vi "qtest.vi"() -> ()   [LabVIEW 2020]
uses:
  5df3b76d-11be-4eb4-bfe8-7a0dabd50acf.vi
  7e36f1bc-8072-43ef-9e73-c82577f060f5.vi
panel:
  out "x-y":u32
  out "Elemente 5":cluster{"Numerisch":dbl, "Numerisch 2":dbl}[](array[cluster])
  out "Elemente 4":cluster{"Numerisch":dbl, "Numerisch 2":dbl}[](array[cluster])
  out "Elemente 3":cluster{"Numerisch":dbl, "Numerisch 2":dbl}[](array[cluster])
  in  "Stopp":bool
  out "Elemente 2":cluster{"Numerisch":dbl, "Numerisch 2":dbl}[](array[cluster])
  out "Elemente":cluster{"Numerisch":dbl, "Numerisch 2":dbl}[](array[cluster])
  in  "Cluster":cluster{"Numerisch":dbl, "Numerisch 2":dbl}
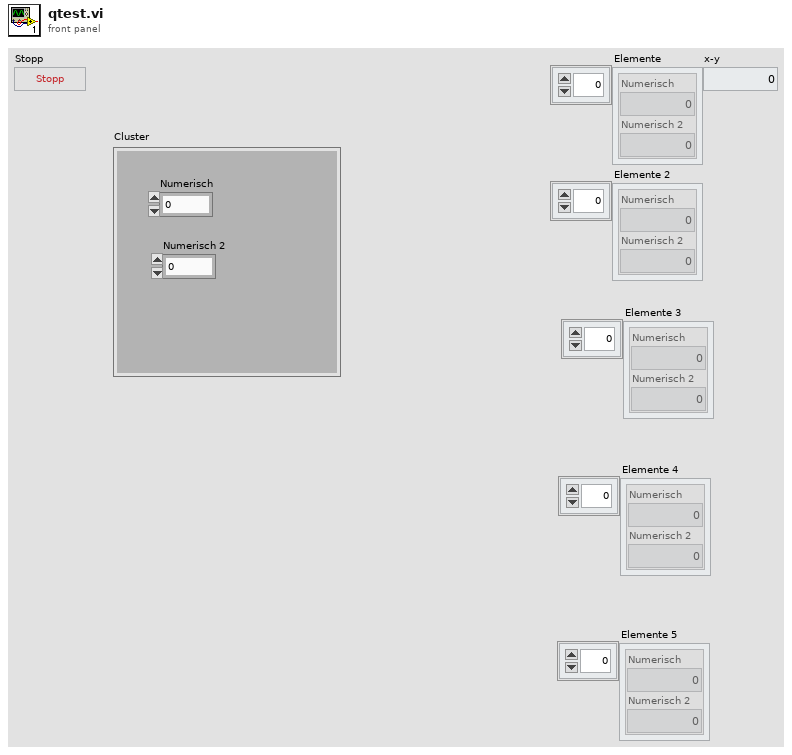
[diagram p1: front panel]
types:
  T1 = cluster{"number: 0 to 1":dbl, "number: 0 to 1":dbl}
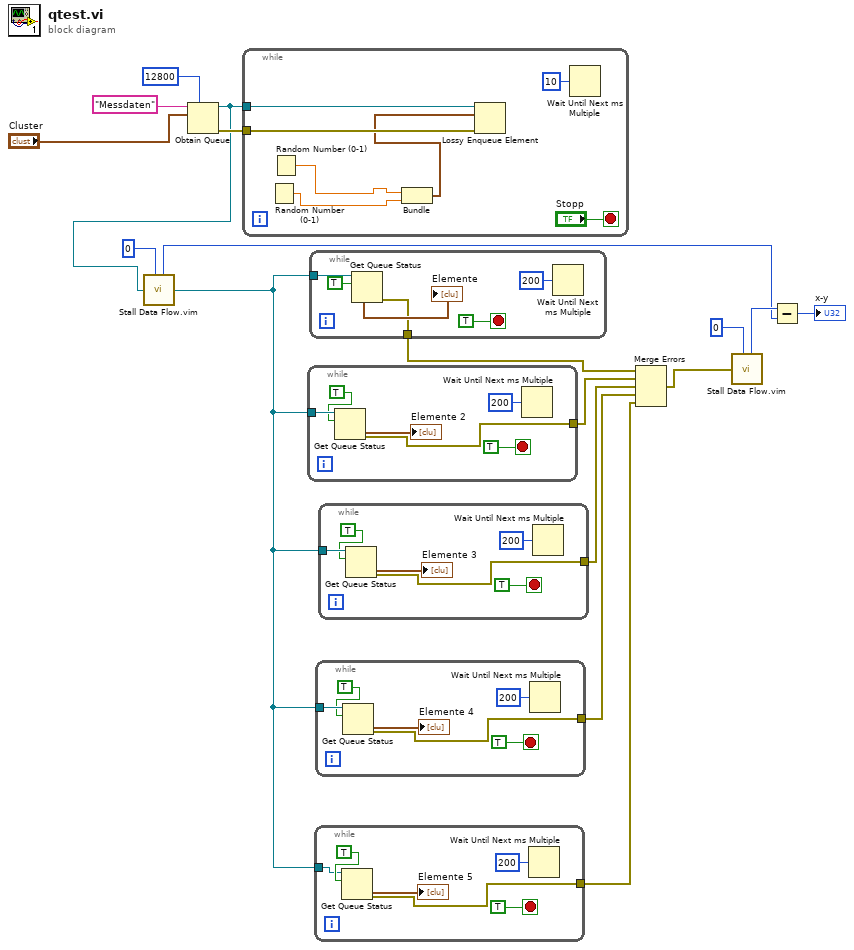
[diagram p0: block diagram]
diagram:
  n1 = Obtain Queue(max queue size (-1, unlimited)=12800 ("Maximale Queue-Größe (-1, unbegrenzt)"), name (unnamed)="Messdaten" ("Name (unbenannt)"), element data type="Cluster") -> (queue out=w8:refnum<queue>, error out=w15:errorcluster)  [unwired: 2 in, 1 out]
  n2 = call "Stall Data Flow.vim"("value in"=w8, "milliseconds to wait"=u32 0) -> ("millisecond timer value"=w2:u32, "value out"=w7:refnum<queue>)
  n3 = while {
    tunnel: w8 -> [w24]
    tunnel: w15 -> [w23]
    stop <- "Stopp" stop-if-true
    n4 = Random Number (0-1)() -> (number: 0 to 1=w21:dbl)
    n5 = Random Number (0-1)() -> (number: 0 to 1=w20:dbl)
    n6 = Bundle("number: 0 to 1"=w20, "number: 0 to 1"=w21) -> (w19:T1)  [unwired: 1 in]
    n7 = Lossy Enqueue Element(queue=w24, element=w19, error in (no error)=w23) -> ()  [unwired: 4 out]
    n8 = Wait Until Next ms Multiple(millisecond multiple=u32 10 ("ms")) -> ()  [unwired: 1 out]
  }
  n9 = while {
    tunnel: w7 -> [w30]
    tunnel: [w25] -> w13
    stop <- TRUE stop-if-true
    n10 = Get Queue Status(queue=w30, return elements? (F)=TRUE ("Elemente ausgeben? (F)")) -> (error out=w25:errorcluster, elements=→"Elemente 2":cluster{"Numerisch":dbl, "Numerisch 2":dbl}[])  [unwired: 1 in, 6 out]
    n11 = Wait Until Next ms Multiple(millisecond multiple=u32 200 ("ms")) -> ()  [unwired: 1 out]
  }
  n12 = while {
    tunnel: w7 -> [w35]
    tunnel: [w31] -> w12
    stop <- TRUE stop-if-true
    n13 = Get Queue Status(queue=w35, return elements? (F)=TRUE ("Elemente ausgeben? (F)")) -> (error out=w31:errorcluster, elements=→"Elemente":cluster{"Numerisch":dbl, "Numerisch 2":dbl}[])  [unwired: 1 in, 6 out]
    n14 = Wait Until Next ms Multiple(millisecond multiple=u32 200 ("ms")) -> ()  [unwired: 1 out]
  }
  n15 = while {
    tunnel: [w38] -> w9
    tunnel: w7 -> [w37]
    stop <- TRUE stop-if-true
    n16 = Get Queue Status(queue=w37, return elements? (F)=TRUE ("Elemente ausgeben? (F)")) -> (error out=w38:errorcluster, elements=→"Elemente 5":cluster{"Numerisch":dbl, "Numerisch 2":dbl}[])  [unwired: 1 in, 6 out]
    n17 = Wait Until Next ms Multiple(millisecond multiple=u32 200 ("ms")) -> ()  [unwired: 1 out]
  }
  n18 = while {
    tunnel: w7 -> [w48]
    tunnel: [w43] -> w10
    stop <- TRUE stop-if-true
    n19 = Get Queue Status(queue=w48, return elements? (F)=TRUE ("Elemente ausgeben? (F)")) -> (error out=w43:errorcluster, elements=→"Elemente 4":cluster{"Numerisch":dbl, "Numerisch 2":dbl}[])  [unwired: 1 in, 6 out]
    n20 = Wait Until Next ms Multiple(millisecond multiple=u32 200 ("ms")) -> ()  [unwired: 1 out]
  }
  n21 = while {
    tunnel: w7 -> [w54]
    tunnel: [w49] -> w11
    stop <- TRUE stop-if-true
    n22 = Get Queue Status(queue=w54, return elements? (F)=TRUE ("Elemente ausgeben? (F)")) -> (error out=w49:errorcluster, elements=→"Elemente 3":cluster{"Numerisch":dbl, "Numerisch 2":dbl}[])  [unwired: 1 in, 6 out]
    n23 = Wait Until Next ms Multiple(millisecond multiple=u32 200 ("ms")) -> ()  [unwired: 1 out]
  }
  n24 = Merge Errors(w12, w13, w11, w10, w9) -> (w6:errorcluster)
  n25 = call "Stall Data Flow.vim"("value in"=w6, "milliseconds to wait"=u32 0) -> ("millisecond timer value"=w3:u32)  [unwired: 1 out]
  n26 = Subtract(x=w3, y=w2) -> (x-y=→"x-y":u32)
